vi "Express VI - Sample Compression.vi"() -> ()   [LabVIEW 2023]
doc: "Demonstrates the use of the Sample Compression Express VI."
panel:
  out "Signal Chart":dynamicdata(graph)
  # "Overview: Demonstrates the use of the Sample Compression Express VI.\nInstructions:\n1. Run the VI.\n2. The Sine with Noise plot contains 100 samples.\n3. The Sine with Noise (Max) plot is the result of Sample Compression, configured with a reduction factor of 10 and a reduction method of Maximum.\n4. Open the block diagram. Right-click on the Sample Compression Express VI and select Properties from the menu.\n5. Experiment with the other configuration options for the Sample Compression Express VI."
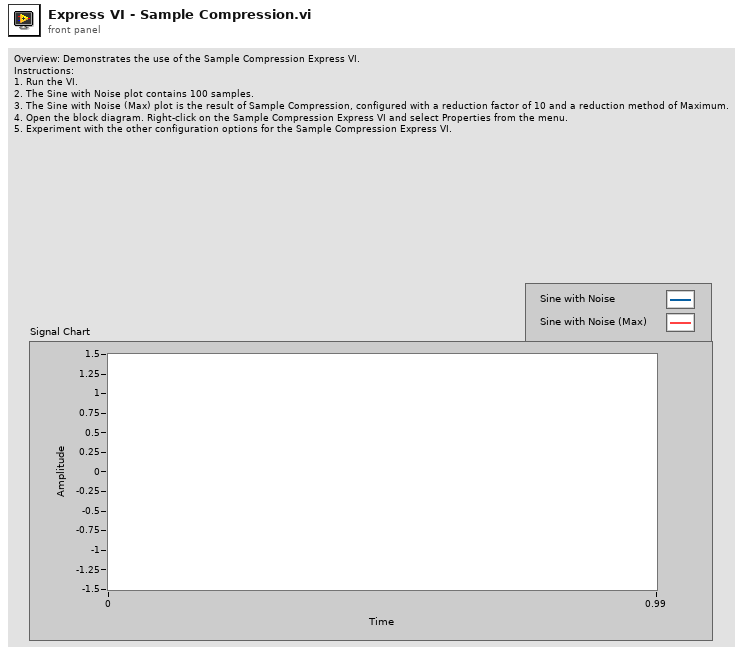
[diagram p1: front panel]
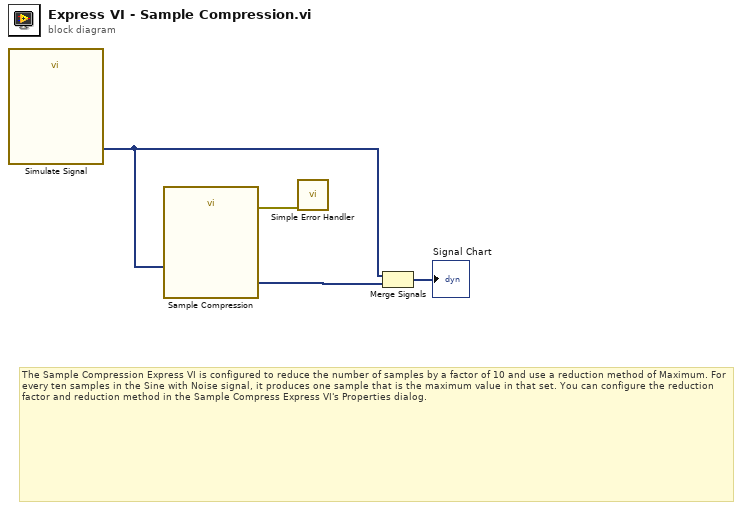
[diagram p0: block diagram]
diagram:
  # "The Sample Compression Express VI is configured to reduce the number of samples by a factor of 10 and use a reduction method of Maximum. For every ten samples in the Sine with Noise signal, it produces one sample that is the maximum value in that set. You can configure the reduction factor and reduction method in the Sample Compress Express VI's Properties dialog."
  n1 = call "Simulate Signal"() -> ("Sine with Noise"=w4:dynamicdata)  [unwired: 14 in, 1 out]
  n2 = call "Sample Compression"("Signals"=w4) -> ("error out"=w1:errorcluster, "Maximum"=w2:dynamicdata)  [unwired: 8 in, 1 out]
  n3 = call <vilib>:"Simple Error Handler.vi"("error in (no error)"=w1) -> ()  [unwired: 4 in, 5 out]
  n4 = Merge Signals(w4, w2) -> (→"Signal Chart":dynamicdata)
